vi "Methods.vi"(7 "error in":errorcluster) -> (3 "Methods":string[](array[string]), 5 "error out":errorcluster)   [LabVIEW 2012]
uses:
  Folders.ctl
  Design Server.lvlib
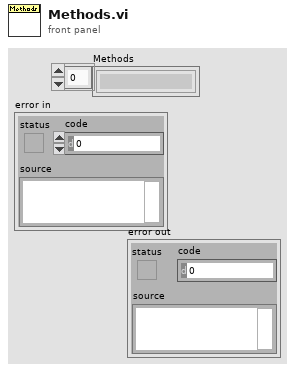
[diagram p1: front panel]
types:
  T1 = typedef "Design Server.lvlib/Folders.ctl" = enum16{"MathcadMethods", "RequestedDesigns", "CompletedDesigns", "MathcadCode", "CollabnetSVN.exe"}
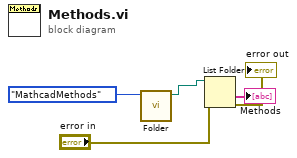
[diagram p0: block diagram]
diagram:
  n1 = call "Folder.vi"("Folders"=Folders."MathcadMethods") -> ("FolderPath"=w4:path)  [unwired: 8 in, 2 out]
  n2 = List Folder(path=w4, error in="error in") -> (folder names=→"Methods":string[], error out=→"error out":errorcluster)  [unwired: 2 in, 2 out]
